vi "Read Line.vi"(8 "error in (no error)":errorcluster, 11 "Set Output Line Msg in":refnum<class "Set Output Line Msg.lvclass">) -> (0 "error out":errorcluster, 2 "Line":i32, 3 "Set Output Line Msg out":refnum<class "Set Output Line Msg.lvclass">)   [LabVIEW 2017, in "BNT_DAQmx.lvlib" / "Set Output Line Msg.lvclass"]
uses:
  Set Output Line Msg.lvclass
  Set Output Line Msg.lvclass/Set Output Line Msg.ctl
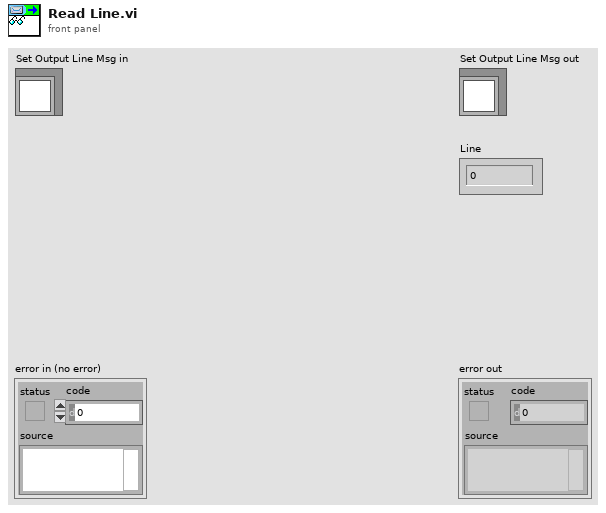
[diagram p1: front panel]
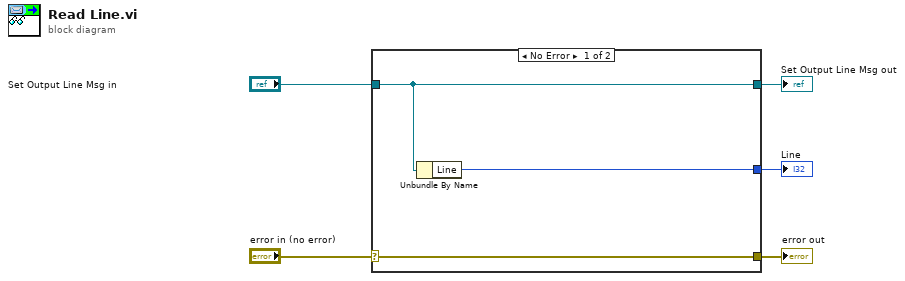
[diagram p0: block diagram]
diagram:
  n1 = case shown="No Error" "error in (no error)" {
    selector: "error in (no error)" -> [w8 w9]
    tunnel: [w8 w9] -> w4
    tunnel: [w7 w10] -> w2
    tunnel: "Set Output Line Msg in" -> [w7 w10]
    tunnel: [w6 _] -> w1
    frame No Error {
      n2 = Unbundle By Name(w7) -> ("Line"=w6:i32)
    }
    frame Error {
    }
  }
  "error out" <- w4
  "Set Output Line Msg out" <- w2
  "Line" <- w1
